vi "Update Fire.vi"(8 "error in (no error)":errorcluster, 10 "Fire":dbl format="%.2f C°", 11 "Cooker Actor in":refnum<class "Cooker Actor.lvclass">) -> (0 "error out":errorcluster, 3 "Cooker Actor out":refnum<class "Cooker Actor.lvclass">)   [LabVIEW 2024, in "Cooker Actor.lvlib" / "Cooker Actor.lvclass"]
uses:
  Cooker Actor.lvclass
  Cooker Actor.lvclass/Cooker Actor.ctl
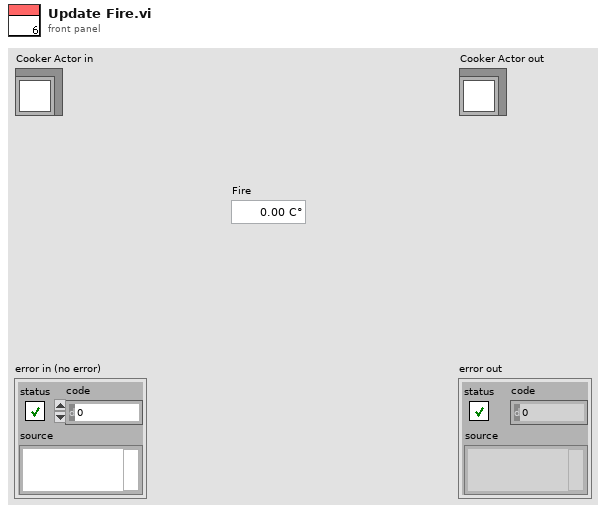
[diagram p1: front panel]
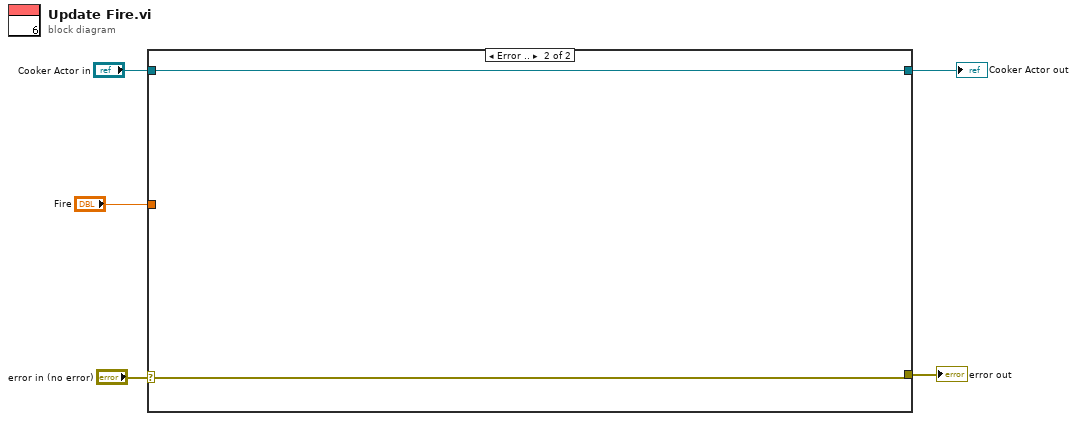
[diagram p0: block diagram]
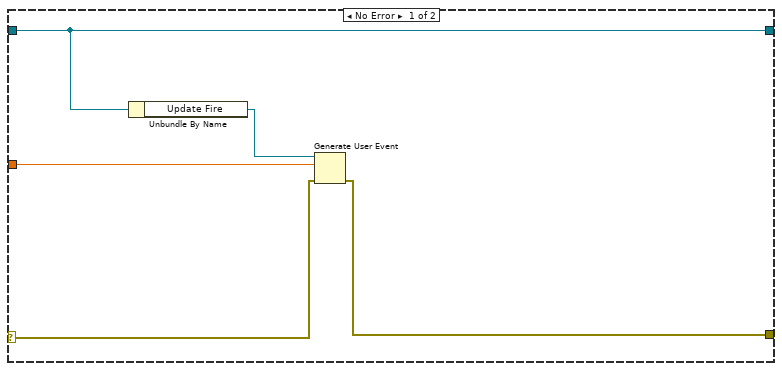
[diagram p2: hidden frame]
diagram:
  n1 = case shown="Error .." "error in (no error)" {
    selector: "error in (no error)" -> [w7 w12]
    tunnel: [w10 w11] -> w3
    tunnel: "Cooker Actor in" -> [w10 w11]
    tunnel: "Fire" -> [w8 _]
    tunnel: [w6 w12] -> w1
    frame No Error {
      n2 = Unbundle By Name(w10) -> ("Update Fire"=w9:refnum<user-event>)
      n3 = Generate User Event(user event=w9, event data cluster=w8, error in=w7) -> (error out=w6:errorcluster)  [unwired: 1 in, 1 out]
    }
    frame Error {
    }
  }
  "error out" <- w1
  "Cooker Actor out" <- w3
